vi "PRBS signal generator.vi"(5 "Amplitude [deg]":dbl, 6 "Error In":errorcluster, 9 "Highest frequency  \n[Hz, cycles/sec]":i32=2 step=1) -> (0 "error out":errorcluster)   [LabVIEW 2018]
uses:
  <vilib>/addons/System Identification/NI_SysID.lvlib
panel:
  out "x/y":dbl
  out "Signal sampling period [sec]":dbl=100.0
  out "initialized array":dbl[](array[numeric])
  in  "Signal duration [sec]":i64=128 caption="Signal duration"
  out "Sampled chirp signal":dbl[](array[numeric])
  out "Chirp signal":dbl[](graph)
  # "INPUTS"
  # "OUTPUTS"
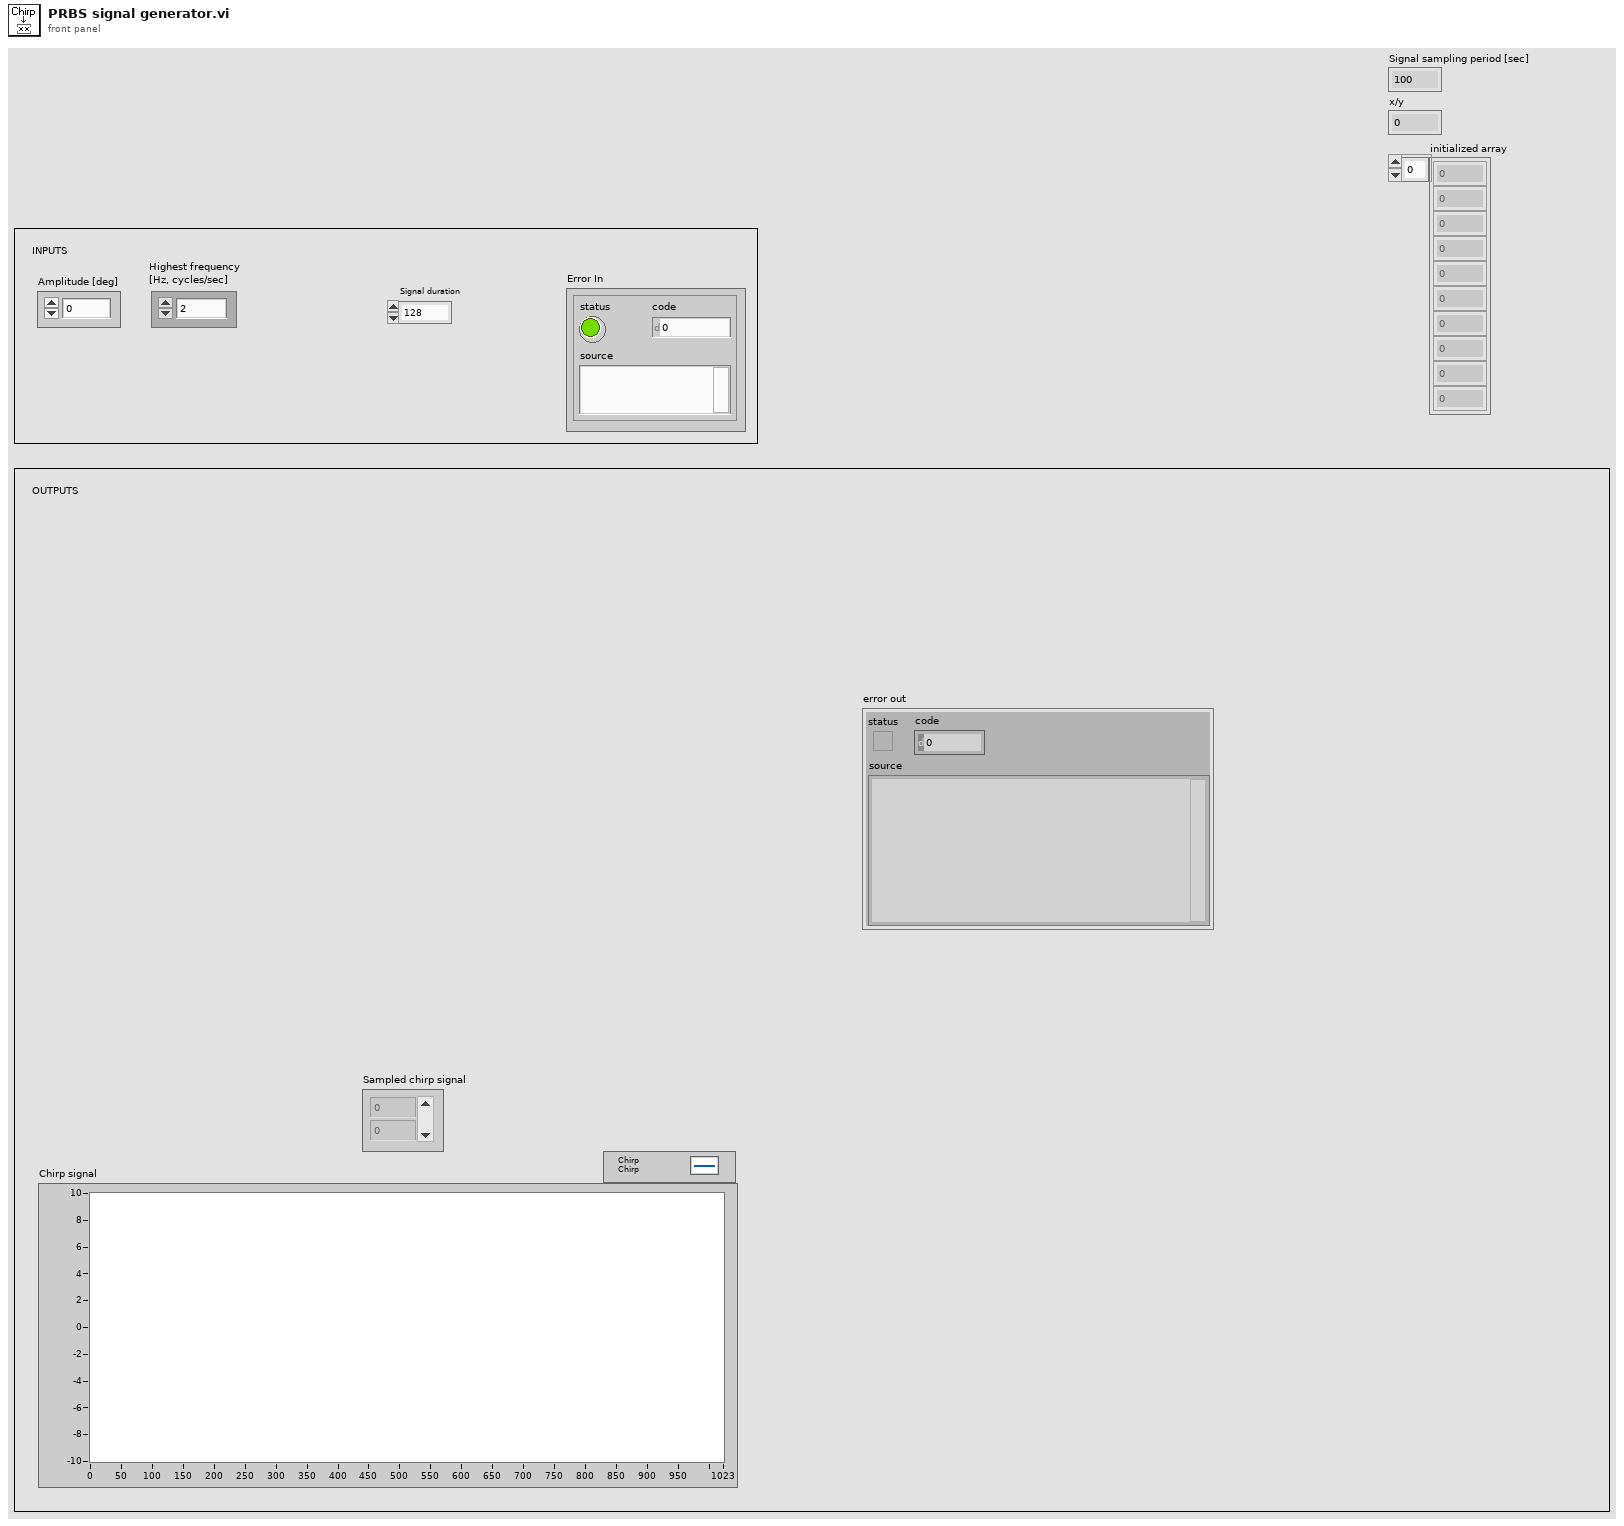
[diagram p1: front panel]
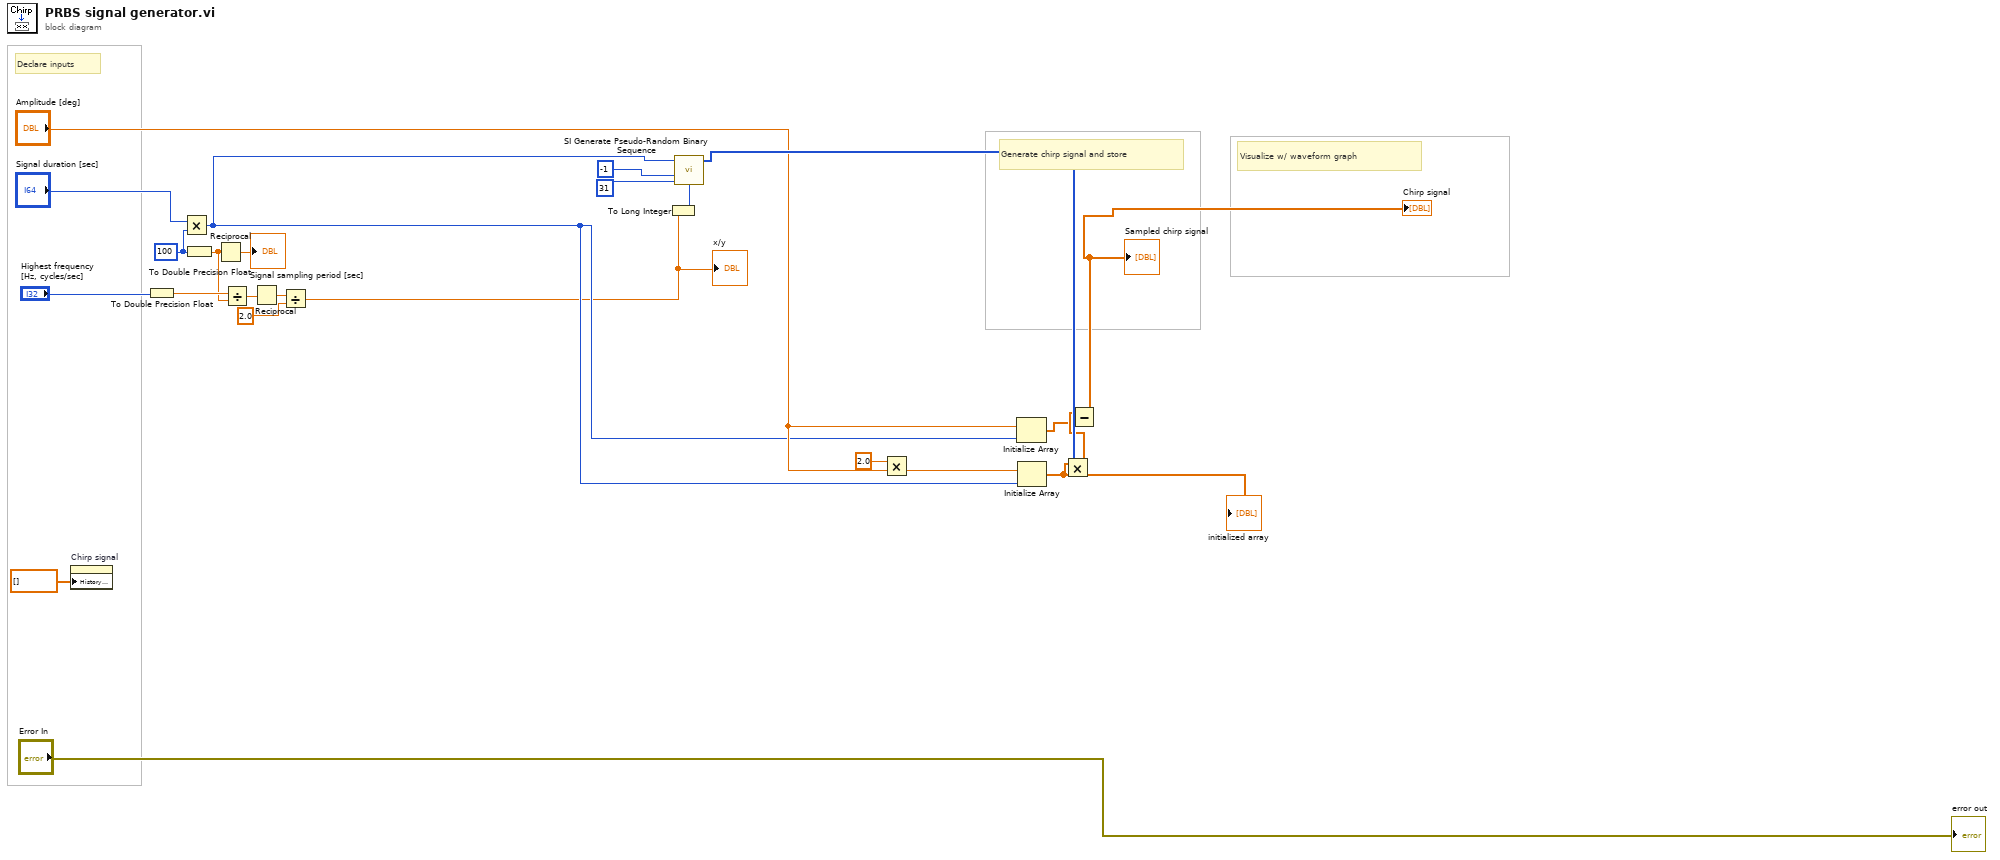
[diagram p0: block diagram]
diagram:
  w12 = i64 100 ("y")
  # "Generate chirp signal and store"
  # "Visualize w/ waveform graph"
  # "Declare inputs"
  n1 = property on="Chirp signal" class="WFChart (strict)"("History Data"=dbl[] []) -> ()  [unwired: 2 in, 2 out]
  n2 = To Double Precision Float(number="Highest frequency  \n[Hz, cycles/sec]") -> (double precision float=w9:dbl)
  n3 = Multiply(x="Signal duration [sec]", y=w12) -> (x*y=w13:i64)
  n4 = To Double Precision Float(number=w12) -> (double precision float=w8:dbl)
  n5 = Reciprocal(x=w8) -> (1/x=→"Signal sampling period [sec]":dbl)
  n6 = Divide(x=w9, y=w8) -> (x/y=w7:dbl)
  n7 = Reciprocal(x=w7) -> (1/x=w6:dbl)
  n8 = Divide(x=w6, y=2.0) -> (x/y=w4:dbl)
  "x/y" <- w4
  n9 = To Long Integer(number=w4) -> (32bit integer=w3:i32)
  n10 = call <vilib>:"SI Generate Pseudo-Random Binary Sequence.vi"("upsampling factor"=w3, "seed"=i64 -1, "polynomial order"=31, "samples"=w13) -> ("PRBS"=w22:u8[])  [unwired: 7 in]
  n11 = Multiply(x=2.0, y="Amplitude [deg]") -> (x*y=w20:dbl)
  n12 = Initialize Array("Amplitude [deg]", w13) -> (w14:dbl[])
  n13 = Initialize Array(w20, w13) -> (w21:dbl[])
  "initialized array" <- w21
  n14 = Multiply(x=w21, y=w22) -> (x*y=w15:dbl[])
  n15 = Subtract(x=w15, y=w14) -> (x-y=→"Chirp signal" →"Sampled chirp signal":dbl[])
  "error out" <- "Error In"
